vi "Phasor Compute 1-Exp Gate Array v2.vi"(8 "Error In":errorcluster, 9 "Gates Definitions":T3={"First Gate: t1"=0.0, "Gate Width: W"=0.0, "Gate Step: d"=0.0, "# Gates: G"=0.0, "Use Gate Center"=FALSE, "Frames/Image: F"=50, "Gates/Frame: L"=0, "Bits/Frame: q"=0, "Multiplicity: p"=0, "Gate Type"=enum."Square", "Gate Edge s"=4.0, "Gate Top Slope"=4.0, "Reversed Sawtooth?"=FALSE, "Computation"=FALSE, "User-defined Gate"={"X Array"=[], "Y Array"=[]}, "Tolerance"=50.0, "Integration"=enum."Item 0", "# Steps"=50.0, "Type of User-defined Function"=enum."Gate"}, 11 "Decay Definition":T1={"offset: t0"=0.0, "period: T"=0.0, "lifetime: tau"=0.0, "Incident Signal: I"=0.5, "Normalized Decays"=FALSE, "IRF Model"=enum."Dirac", "IRF Parameter 1"=0.0, "Poisson Signal"=FALSE}) -> (0 "Error Out":errorcluster, 1 "Gate Image Array":ext[](array[numeric]), 3 "t Array":ext[](array[numeric]), 4 "Small Gate Values?":bool, 6 "CPU (s)":dbl)   [LabVIEW 2021, in "Phasor.lvlib"]
uses:
  Phasor.lvlib
  Phasor Gate Definitions.ctl
  Phasor Gate Type.ctl
  Graphs/XY Graph/XY Plot Data.ctl
  Phasor Decay Definiton.ctl
  Phasor IRF Model.ctl
  Phasor Photon-Counting Saturation Parameters.ctl
  Arrays/Linear Ramp End Options.ctl
  Phasor Gate & Decay Parameters.ctl
  c327f329-df48-4cbd-af17-0505137efb44.vi
  19793270-9f6f-421c-b0b4-4a6df58db2d8.vi
  bce56a49-f57b-428e-8cfb-829b6e224b2d.vi
  9dc9122e-8396-4e29-9b52-206296392f6e.vi
  09e65239-3f09-4922-a97b-00e12ebb298a.vi
  a4873a35-ead0-464d-8454-7d3b7b3dc21e.vi
  430a8be0-ec63-490d-ae91-6adec514d333.vi
  bfad809a-910b-4a1f-913e-0342548baa46.vi
  822bd012-03ef-446a-9035-c62730970759.vi
  9329e439-e603-4ca8-9979-680bb8b82628.vi
  12aa5bdc-9085-4c22-9899-1a2d30a0f259.vi
  2b2e435f-01ea-4379-bbb3-bd43ea243b44.vi
  e19b1486-ca4b-43fe-9b82-4ecd58cc5538.vi
  9dc9122e-8396-4e29-9b52-206296392f6e.vi/8a80743f-1319-44c8-96b0-3ef8fc688731.vi
  9dc9122e-8396-4e29-9b52-206296392f6e.vi/931f4f8f-d8c6-4056-833f-5c8fe97b24b9.vi
  09e65239-3f09-4922-a97b-00e12ebb298a.vi/8a80743f-1319-44c8-96b0-3ef8fc688731.vi
  09e65239-3f09-4922-a97b-00e12ebb298a.vi/931f4f8f-d8c6-4056-833f-5c8fe97b24b9.vi
  430a8be0-ec63-490d-ae91-6adec514d333.vi/8a80743f-1319-44c8-96b0-3ef8fc688731.vi
  430a8be0-ec63-490d-ae91-6adec514d333.vi/931f4f8f-d8c6-4056-833f-5c8fe97b24b9.vi
  9329e439-e603-4ca8-9979-680bb8b82628.vi/8a80743f-1319-44c8-96b0-3ef8fc688731.vi
  9329e439-e603-4ca8-9979-680bb8b82628.vi/931f4f8f-d8c6-4056-833f-5c8fe97b24b9.vi
  2b2e435f-01ea-4379-bbb3-bd43ea243b44.vi/8a80743f-1319-44c8-96b0-3ef8fc688731.vi
  2b2e435f-01ea-4379-bbb3-bd43ea243b44.vi/931f4f8f-d8c6-4056-833f-5c8fe97b24b9.vi
  Phasor Abort Parallel Computation.vi
  Arrays/Arrays.lvlib
  Graphs/XY Graph/XY Graph Add-Ons.lvlib
  Time/Time.lvlib
panel:
  out "XY Graph":cluster{ext[], ext[]}[](graph)
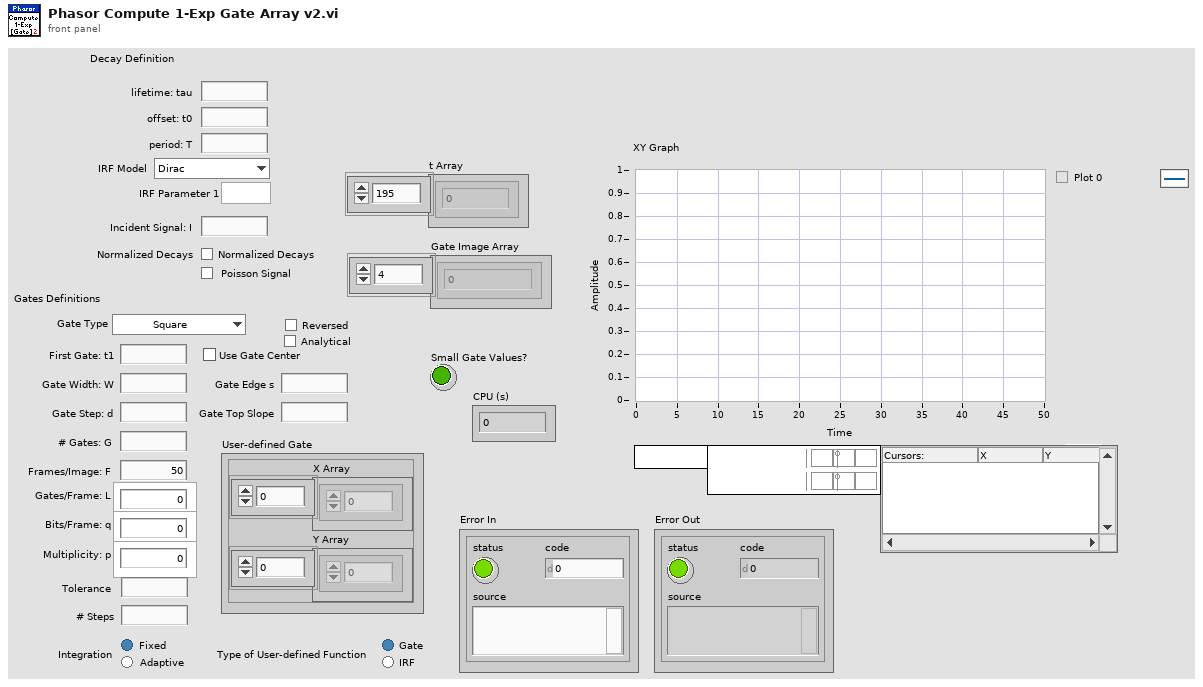
[diagram p1: front panel]
types:
  T1 = typedef "Phasor.lvlib/Phasor Decay Definiton.ctl" = cluster{"offset: t0":ext, "period: T":ext, "lifetime: tau":ext, "Incident Signal: I":ext, "Normalized Decays":bool, "IRF Model":T2, "IRF Parameter 1":ext, "Poisson Signal":bool}
  T2 = typedef "Phasor.lvlib/Phasor IRF Model.ctl" = enum16{"Dirac", "Exponential"}
  T3 = typedef "Phasor.lvlib/Phasor Gate Definitions.ctl" = cluster{"First Gate: t1":ext, "Gate Width: W":ext, "Gate Step: d":ext, "# Gates: G":ext, "Use Gate Center":bool, "Frames/Image: F":i32, "Gates/Frame: L":i32, "Bits/Frame: q":i32, "Multiplicity: p":i32, "Gate Type":T4, "Gate Edge s":ext, "Gate Top Slope":ext, "Reversed Sawtooth?":bool, "Computation":bool, "User-defined Gate":T5, "Tolerance":ext, "Integration":enum32{"Item 0", "Item 1"}, "# Steps":ext, "Type of User-defined Function":enum32{"Gate", "IRF"}}
  T4 = typedef "Phasor.lvlib/Phasor Gate Type.ctl" = enum16{"Square", "Finite Edge Square", "Finite Edge, Tilted Top Square", "Triangle", "Sawtooth", "User-defined"}
  T5 = typedef "XY Graph Add-Ons.lvlib/XY Plot Data.ctl" = cluster{"X Array":dbl[], "Y Array":dbl[]}
  T6 = typedef "Phasor.lvlib/Phasor Photon-Counting Saturation Parameters.ctl" = cluster{"Frames/Image: F":i32, "Gates/Frame: L":i32, "Multiplicity: p":i32, "Bits/Frame: q":i32}
  T7 = typedef "Phasor.lvlib/Phasor Gate & Decay Parameters.ctl" = cluster{"W":dbl, "T":dbl, "tau":dbl, "t_0":dbl, "Gate Type":T4, "t_i":dbl, "sR":dbl, "sF":dbl, "s":dbl, "Reversed Sawtooth":bool, "IRF Model":T2, "IRF Parameter 1":dbl, "User-defined Gate":T5, "Type of User-defined Function":enum32{"Gate", "IRF"}, "A":dbl}
  T8 = typedef "Arrays.lvlib/Linear Ramp End Options.ctl" = enum16{"Include Min/Exclude Max", "Exclude Min/Include Max", "Include Both Ends", "Exclude Both Ends"}
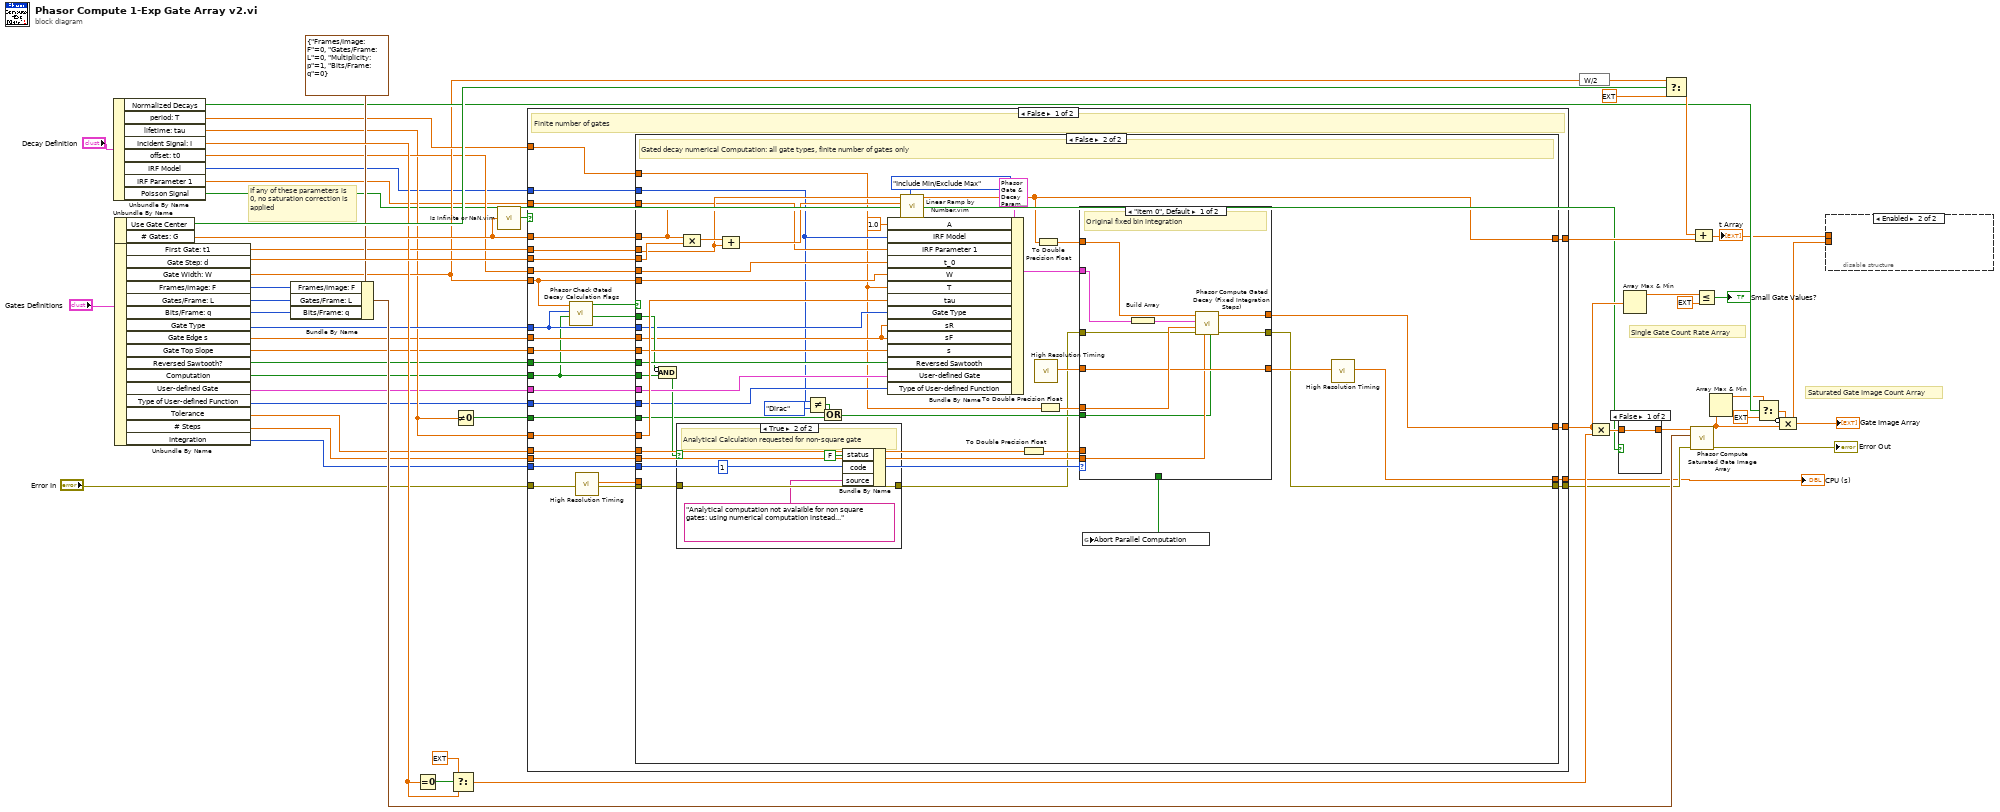
[diagram p0: block diagram]
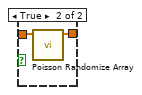
[diagram p2: hidden frame]
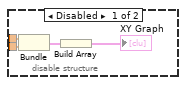
[diagram p3: hidden frame]
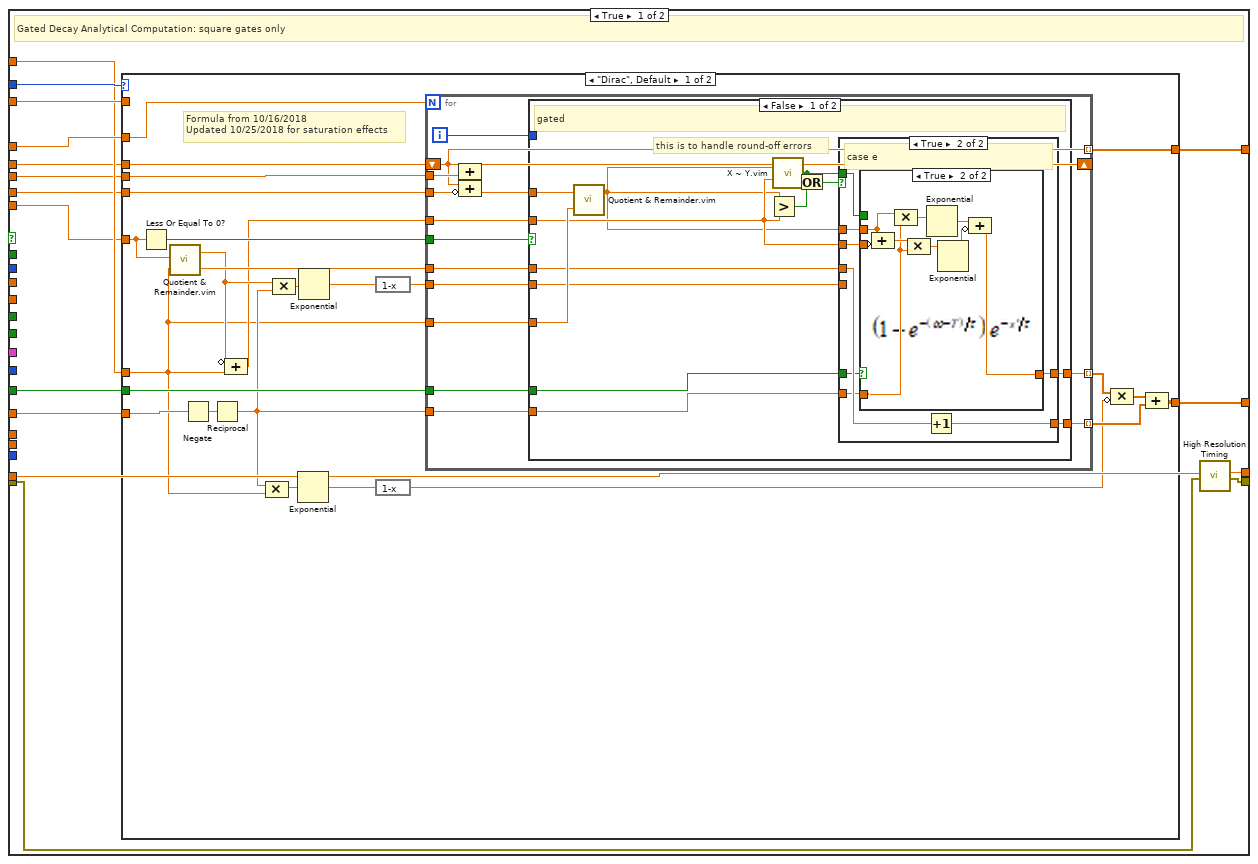
[diagram p4: hidden frame]
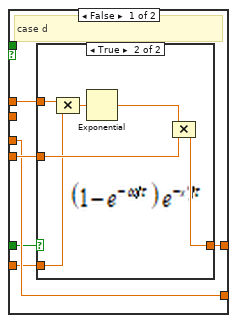
[diagram p5: hidden frame]
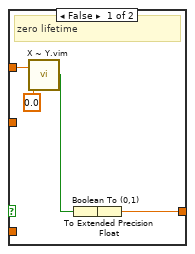
[diagram p6: hidden frame]
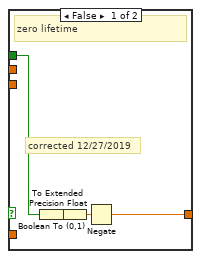
[diagram p7: hidden frame]
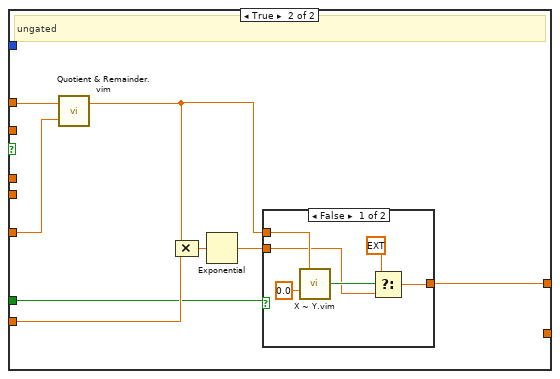
[diagram p8: hidden frame]
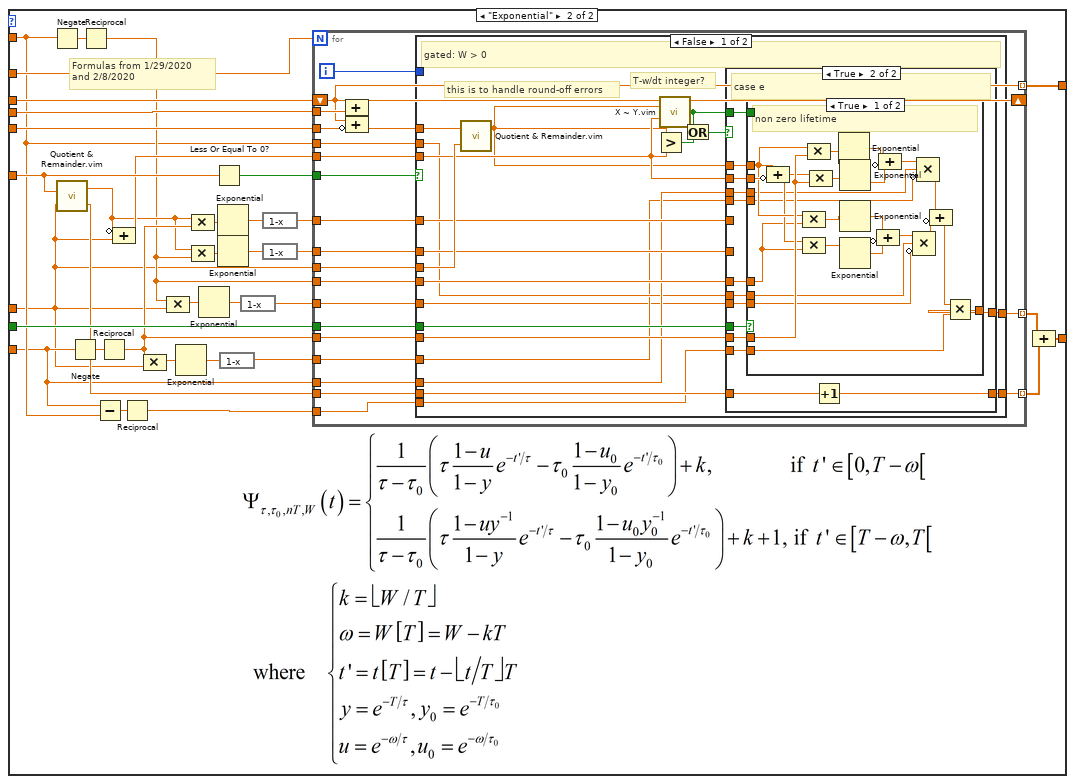
[diagram p10: hidden frame]
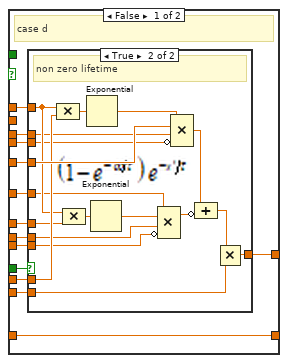
[diagram p11: hidden frame]
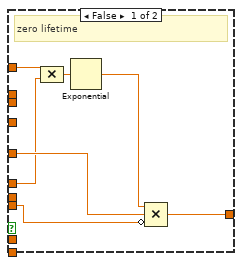
[diagram p12: hidden frame]
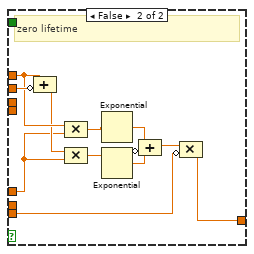
[diagram p13: hidden frame]
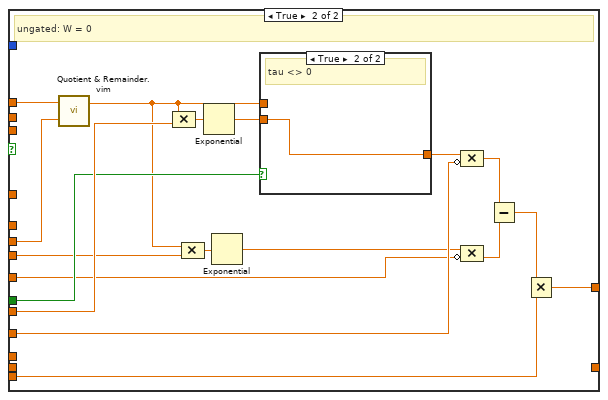
[diagram p14: hidden frame]
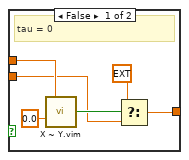
[diagram p15: hidden frame]
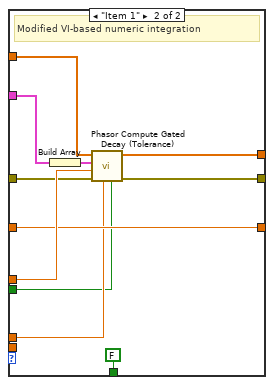
[diagram p16: hidden frame]
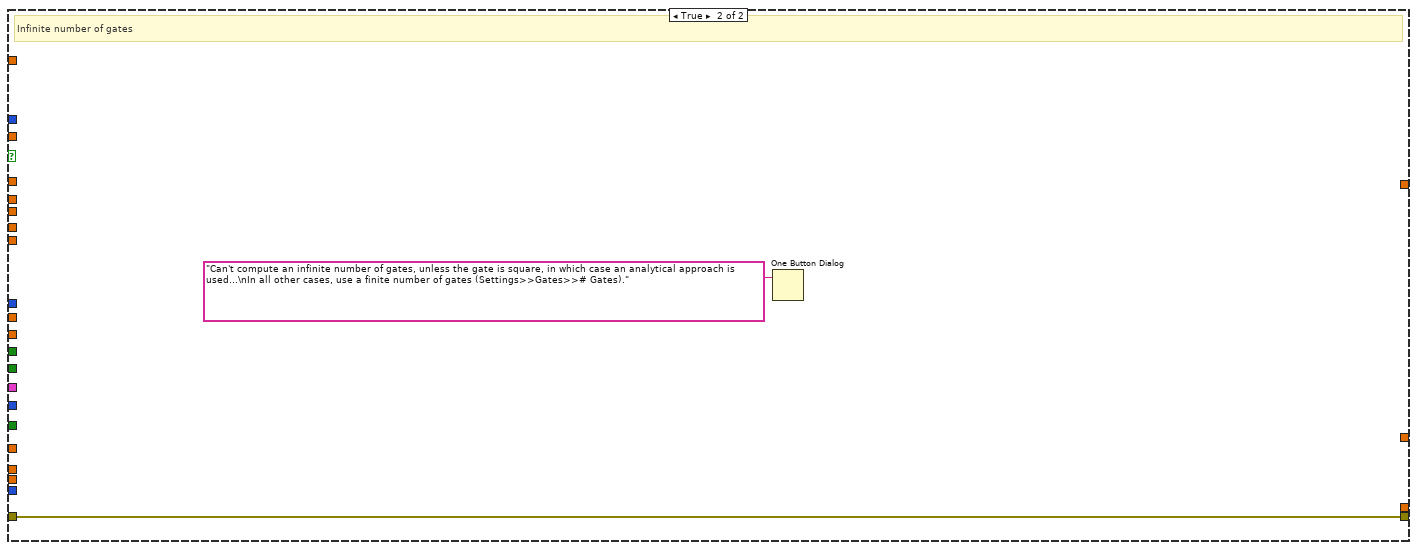
[diagram p18: hidden frame]
diagram:
  # "If any of these parameters is 0, no saturation correction is applied"
  # "Saturated Gate Image Count Array"
  # "Single Gate Count Rate Array"
  n1 = Unbundle By Name("Decay Definition") -> ("Normalized Decays"=w36:bool, "period: T"=w32:ext, "lifetime: tau"=w23:ext, "Incident Signal: I"=w44:ext, "offset: t0"=w27:ext, "IRF Model"=w11:T2, "IRF Parameter 1"=w10:ext, "Poisson Signal"=w1:bool)
  n2 = Unbundle By Name("Gates Definitions") -> ("Use Gate Center"=w48:bool, "# Gates: G"=w49:ext)
  n3 = Unbundle By Name("Gates Definitions") -> ("First Gate: t1"=w33:ext, "Gate Step: d"=w55:ext, "Gate Width: W"=w28:ext, "Frames/Image: F"=w43:i32, "Gates/Frame: L"=w42:i32, "Bits/Frame: q"=w41:i32, "Gate Type"=w26:T4, "Gate Edge s"=w21:ext, "Gate Top Slope"=w20:ext, "Reversed Sawtooth?"=w16:bool, "Computation"=w12:bool, "User-defined Gate"=w9:T5, "Type of User-defined Function"=w4:enum32{"Gate", "IRF"}, "Tolerance"=w8:ext, "# Steps"=w5:ext, "Integration"=w6:enum32{"Item 0", "Item 1"})
  n4 = Bundle By Name(cluster=T6 {"Frames/Image: F"=0, "Gates/Frame: L"=0, "Multiplicity: p"=1, "Bits/Frame: q"=0} ("Saturation Parameters"), "Frames/Image: F"=w43, "Gates/Frame: L"=w42, "Bits/Frame: q"=w41) -> (w40:T6)
  n5 = Equal To 0?(x=w44) -> (x = 0?=w45:bool)
  n6 = Select(t=ext 1.0, s=w45, f=w44) -> (s? t:f=w46:ext)
  n7 = Not Equal To 0?(x=w23) -> (x != 0?=w22:bool)
  n8 = call "Is Infinite or NaN.vim"("Number"=w49) -> ("Is NaN or Inf?"=w13:bool)  [unwired: 8 in]
  n9 = case shown="False" w13 {
    tunnel: w26 -> [w70 _]
    tunnel: w33 -> [w84 _]
    tunnel: w55 -> [w83 _]
    tunnel: w27 -> [w82 _]
    tunnel: w32 -> [w81 _]
    tunnel: w23 -> [w80 _]
    tunnel: [w79 _] -> w25
    tunnel: [w78 _] -> w24
    tunnel: w22 -> [w77 _]
    tunnel: w21 -> [w76 _]
    tunnel: w20 -> [w75 _]
    tunnel: w16 -> [w74 _]
    tunnel: w49 -> [w73 _]
    tunnel: w28 -> [w63 _]
    tunnel: "Error In" -> [w71 w467]
    tunnel: [w72 w467] -> w14
    tunnel: w12 -> [w65 _]
    tunnel: w11 -> [w69 _]
    tunnel: w10 -> [w68 _]
    tunnel: w9 -> [w67 _]
    tunnel: w8 -> [w66 _]
    tunnel: [w62 _] -> w7
    tunnel: w6 -> [w59 _]
    tunnel: w5 -> [w58 _]
    tunnel: w4 -> [w57 _]
    frame False {
      # "Finite number of gates"
      n10 = call "Phasor Check Gated Decay Calculation Flags.vi"("Analytical Computation?"=w65, "Gate/IRF Type"=w70, "Gate Width: W"=w63) -> ("Square Gate?"=w56:bool, "Analytical?"=w64:bool)  [unwired: 7 in]
      n11 = call "High Resolution Timing.vi"("Error In"=w71) -> ("elapsed (relative) seconds"=w60:dbl, "Error Out"=w61:errorcluster)  [unwired: 16 in, 1 out]
      n12 = case shown="False" w64 {
        tunnel: w73 -> [w94 w435]
        tunnel: w84 -> [w88 w432]
        tunnel: w83 -> [w89 w433]
        tunnel: w82 -> [w90 w415]
        tunnel: w63 -> [w91 w411]
        tunnel: w81 -> [w92 w402]
        tunnel: w80 -> [w93 w434]
        tunnel: [w100 w430] -> w78
        tunnel: [w99 w431] -> w79
        tunnel: w77 -> [w98 w416]
        tunnel: w76 -> [_ w413]
        tunnel: w75 -> [_ w429]
        tunnel: w74 -> [_ w428]
        tunnel: [w87 w397] -> w72
        tunnel: w61 -> [w97 w424]
        tunnel: w70 -> [_ w412]
        tunnel: w69 -> [w96 w404]
        tunnel: w68 -> [w95 w427]
        tunnel: w67 -> [_ w426]
        tunnel: w66 -> [_ w425]
        tunnel: w65 -> [_ w423]
        tunnel: w56 -> [_ w422]
        tunnel: [w85 w406] -> w62
        tunnel: w60 -> [w86 _]
        tunnel: w59 -> [_ w417]
        tunnel: w58 -> [_ w414]
        tunnel: w57 -> [_ w410]
        frame True {
          # "Gated Decay Analytical Computation: square gates only"
          n13 = case shown="\"Dirac\", Default" w96 {
            tunnel: w94 -> [w125 w241]
            tunnel: w88 -> [w124 w240]
            tunnel: w89 -> [w123 w239]
            tunnel: w90 -> [w122 w238]
            tunnel: w91 -> [w121 w237]
            tunnel: w92 -> [w101 w207]
            tunnel: w93 -> [w120 w208]
            tunnel: [w119 w236] -> w100
            tunnel: [w118 w235] -> w99
            tunnel: w98 -> [w117 w234]
            tunnel: w95 -> [_ w209]
            frame "Dirac", Default {
              # "Formula from 10/16/2018\nUpdated 10/25/2018 for saturation effects"
              n14 = Less Or Equal To 0?(x=w121) -> (x <= 0?=w106:bool)
              n15 = call "Quotient & Remainder.vim"("y"=w101, "x"=w121) -> ("E(x/y)"=w109:ext, "x - E(x/y)y"=w105:ext)
              n16 = Negate(x=w120) -> (-x=w114:ext)
              n17 = Reciprocal(x=w114) -> (1/x=w104:ext)
              n18 = Compound Arithmetic op=ADD(invert w105, w101) -> (w102:ext)
              n19 = Compound Arithmetic op=MULTIPLY(w104, w101) -> (w113:ext)
              n20 = Compound Arithmetic op=MULTIPLY(w105, w104) -> (w112:ext)
              n21 = Exponential(1:w113) -> (0:w108:ext)
              n22 = Exponential(1:w112) -> (0:w111:ext)
              n23 = expression code="1-x"(w111) -> (w110:ext)
              n24 = expression code="1-x"(w108) -> (w107:ext)
              n25 = for {
                N: w125 -> [_]
                tunnel: w123 -> [w140]
                tunnel: w122 -> [w138]
                tunnel: w101 -> [w136]
                tunnel: w104 -> [w135]
                shift-right: [w139] -> _
                shift-left: w124 -> [w131]
                tunnel: [w131] -> w119 mode=indexing
                tunnel: w110 -> [w134]
                tunnel: w109 -> [w133]
                tunnel: [w127] -> w103 mode=indexing
                tunnel: [w132] -> w116 mode=indexing
                tunnel: w106 -> [w130]
                tunnel: w102 -> [w129]
                tunnel: w117 -> [w128]
                i -> [w126]
                n26 = Compound Arithmetic op=ADD(w131, w140) -> (w139:ext)
                n27 = Compound Arithmetic op=ADD(w131, invert w138) -> (w137:ext)
                n28 = case shown="False" w130 {
                  tunnel: w137 -> [w153 w192]
                  tunnel: w136 -> [w152 w199]
                  tunnel: w135 -> [w146 w198]
                  tunnel: w134 -> [w151 _]
                  tunnel: [w150 w196] -> w127
                  tunnel: w133 -> [w149 _]
                  tunnel: [w148 _] -> w132
                  tunnel: w129 -> [w144 _]
                  tunnel: w128 -> [w145 w193]
                  tunnel: w126 -> [_ _]
                  frame False {
                    # "this is to handle round-off errors"
                    # "gated"
                    n29 = call "Quotient & Remainder.vim"("y"=w152, "x"=w153) -> ("x - E(x/y)y"=w141:ext)  [unwired: 1 out]
                    n30 = Greater?(x=w141, y=w144) -> (0:w147:bool)
                    n31 = call "X ~ Y.vim"("X"=w141, "Y"=w144) -> ("X ~= Y?"=w143:bool)  [unwired: 13 in]
                    n32 = Or(x=w143, y=w147) -> (x .or. y?=w142:bool)
                    n33 = case shown="True" w142 {
                      tunnel: w151 -> [w159 _]
                      tunnel: [w158 w174] -> w150
                      tunnel: w149 -> [w157 w178]
                      tunnel: [w157 w177] -> w148
                      tunnel: w141 -> [w156 w176]
                      tunnel: w146 -> [w155 w175]
                      tunnel: w144 -> [_ w173]
                      tunnel: w145 -> [w154 w172]
                      tunnel: w143 -> [_ w171]
                      frame False {
                        # "case d"
                        n34 = case shown="True" w154 {
                          tunnel: w159 -> [_ w170]
                          tunnel: [w163 w169] -> w158
                          tunnel: w156 -> [w162 w167]
                          tunnel: w155 -> [_ w166]
                          frame False {
                            # "zero lifetime"
                            n35 = call "X ~ Y.vim"("X"=w162, "Y"=0.0) -> ("X ~= Y?"=w160:bool)  [unwired: 13 in]
                            n36 = Boolean To (0,1)(Boolean=w160) -> (0, 1=w164:i16)
                            n37 = To Extended Precision Float(1:w164) -> (0:w163:ext)
                          }
                          frame True {
                            n38 = Compound Arithmetic op=MULTIPLY(w167, w166) -> (w168:ext)
                            n39 = Exponential(1:w168) -> (0:w165:ext)
                            n40 = Compound Arithmetic op=MULTIPLY(w165, w170) -> (w169:ext)
                          }
                        }
                      }
                      frame True {
                        # "case e"
                        n41 = case shown="True" w172 {
                          tunnel: w176 -> [_ w189]
                          tunnel: w175 -> [_ w188]
                          tunnel: [w180 w184] -> w174
                          tunnel: w173 -> [_ w183]
                          tunnel: w171 -> [w179 _]
                          frame False {
                            # "corrected 12/27/2019"
                            # "zero lifetime"
                            n42 = Boolean To (0,1)(Boolean=w179) -> (0, 1=w182:i16)
                            n43 = To Extended Precision Float(1:w182) -> (0:w181:ext)
                            n44 = Negate(x=w181) -> (-x=w180:ext)
                          }
                          frame True {
                            n45 = Compound Arithmetic op=ADD(w189, invert w183) -> (w191:ext)
                            n46 = Compound Arithmetic op=MULTIPLY(w189, w188) -> (w187:ext)
                            n47 = Compound Arithmetic op=MULTIPLY(w191, w188) -> (w190:ext)
                            n48 = Exponential(1:w187) -> (0:w186:ext)
                            n49 = Exponential(1:w190) -> (0:w185:ext)
                            n50 = Compound Arithmetic op=ADD(w186, invert w185) -> (w184:ext)
                          }
                        }
                        n51 = Increment(x=w178) -> (x+1=w177:ext)
                      }
                    }
                  }
                  frame True {
                    # "ungated"
                    n52 = call "Quotient & Remainder.vim"("y"=w199, "x"=w192) -> ("x - E(x/y)y"=w195:ext)  [unwired: 1 out]
                    n53 = Compound Arithmetic op=MULTIPLY(w195, w198) -> (w197:ext)
                    n54 = Exponential(1:w197) -> (0:w194:ext)
                    n55 = case shown="False" w193 {
                      tunnel: [w205 w206] -> w196
                      tunnel: w195 -> [w204 _]
                      tunnel: w194 -> [w200 w206]
                      frame False {
                        n56 = call "X ~ Y.vim"("X"=w204, "Y"=0.0) -> ("X ~= Y?"=w202:bool)  [unwired: 13 in]
                        n57 = Select(t=ext 1.0 ("f"), s=w202, f=w200) -> (s? t:f=w205:ext)
                      }
                      frame True {
                      }
                    }
                  }
                }
              }
              n58 = Compound Arithmetic op=MULTIPLY(w103, invert w107) -> (w115:ext[])
              n59 = Compound Arithmetic op=ADD(w115, w116) -> (w118:ext[])
            }
            frame "Exponential" {
              # "Formulas from 1/29/2020\nand 2/8/2020"
              n60 = Negate(x=w209) -> (-x=w222:ext)
              n61 = call "Quotient & Remainder.vim"("y"=w207, "x"=w237) -> ("E(x/y)"=w227:ext, "x - E(x/y)y"=w214:ext)
              n62 = Negate(x=w208) -> (-x=w232:ext)
              n63 = Reciprocal(x=w222) -> (1/x=w213:ext)
              n64 = Subtract(x=w208, y=w209) -> (x-y=w211:ext)
              n65 = Reciprocal(x=w232) -> (1/x=w224:ext)
              n66 = Compound Arithmetic op=ADD(invert w214, w207) -> (w223:ext)
              n67 = Reciprocal(x=w211) -> (1/x=w210:ext)
              n68 = Compound Arithmetic op=MULTIPLY(w224, w207) -> (w231:ext)
              n69 = Compound Arithmetic op=MULTIPLY(w213, w207) -> (w218:ext)
              n70 = Exponential(1:w231) -> (0:w226:ext)
              n71 = Compound Arithmetic op=MULTIPLY(w214, w224) -> (w230:ext)
              n72 = Compound Arithmetic op=MULTIPLY(w214, w213) -> (w215:ext)
              n73 = Exponential(1:w218) -> (0:w219:ext)
              n74 = Less Or Equal To 0?(x=w237) -> (x <= 0?=w225:bool)
              n75 = Exponential(1:w230) -> (0:w229:ext)
              n76 = Exponential(1:w215) -> (0:w216:ext)
              n77 = expression code="1-x"(w226) -> (w221:ext)
              n78 = expression code="1-x"(w219) -> (w217:ext)
              n79 = expression code="1-x"(w229) -> (w228:ext)
              n80 = expression code="1-x"(w216) -> (w212:ext)
              n81 = for {
                N: w241 -> [_]
                tunnel: w239 -> [w263]
                tunnel: w238 -> [w261]
                tunnel: w207 -> [w259]
                tunnel: w224 -> [w258]
                shift-right: [w262] -> _
                shift-left: w240 -> [w255]
                tunnel: [w255] -> w236 mode=indexing
                tunnel: w228 -> [w257]
                tunnel: w227 -> [w242]
                tunnel: [w244] -> w220 mode=indexing
                tunnel: [w256] -> w233 mode=indexing
                tunnel: w225 -> [w254]
                tunnel: w223 -> [w253]
                tunnel: w234 -> [w252]
                tunnel: w213 -> [w250]
                tunnel: w221 -> [w245]
                tunnel: w217 -> [w249]
                tunnel: w212 -> [w248]
                tunnel: w210 -> [w243]
                tunnel: w209 -> [w247]
                tunnel: w208 -> [w246]
                i -> [w251]
                n82 = Compound Arithmetic op=ADD(w255, w263) -> (w262:ext)
                n83 = Compound Arithmetic op=ADD(w255, invert w261) -> (w260:ext)
                n84 = case shown="False" w254 {
                  tunnel: w260 -> [w283 w388]
                  tunnel: w259 -> [w282 w387]
                  tunnel: w258 -> [w277 w386]
                  tunnel: w257 -> [w281 _]
                  tunnel: w242 -> [w280 _]
                  tunnel: [w279 _] -> w256
                  tunnel: w253 -> [w275 _]
                  tunnel: w252 -> [w276 w383]
                  tunnel: w251 -> [_ _]
                  tunnel: w250 -> [w271 w379]
                  tunnel: w249 -> [w265 w376]
                  tunnel: w248 -> [w270 _]
                  tunnel: w247 -> [w268 _]
                  tunnel: w246 -> [w269 _]
                  tunnel: w245 -> [w267 w381]
                  tunnel: [w266 w371] -> w244
                  tunnel: w243 -> [w264 w372]
                  frame False {
                    # "T-w/dt integer?"
                    # "this is to handle round-off errors"
                    # "gated: W > 0"
                    n85 = call "Quotient & Remainder.vim"("y"=w282, "x"=w283) -> ("x - E(x/y)y"=w272:ext)  [unwired: 1 out]
                    n86 = Greater?(x=w272, y=w275) -> (0:w278:bool)
                    n87 = call "X ~ Y.vim"("X"=w272, "Y"=w275) -> ("X ~= Y?"=w274:bool)  [unwired: 13 in]
                    n88 = Or(x=w274, y=w278) -> (x .or. y?=w273:bool)
                    n89 = case shown="True" w273 {
                      tunnel: w281 -> [w296 _]
                      tunnel: [w295 w331] -> w266
                      tunnel: w280 -> [w294 w335]
                      tunnel: [w294 w334] -> w279
                      tunnel: w272 -> [w293 w333]
                      tunnel: w277 -> [w292 w332]
                      tunnel: w275 -> [_ w330]
                      tunnel: w276 -> [w291 w329]
                      tunnel: w274 -> [_ w328]
                      tunnel: w271 -> [w290 w327]
                      tunnel: w270 -> [w289 _]
                      tunnel: w269 -> [w288 w326]
                      tunnel: w268 -> [w287 w325]
                      tunnel: w267 -> [w286 w324]
                      tunnel: w265 -> [w285 w323]
                      tunnel: w264 -> [w284 w322]
                      frame False {
                        # "case d"
                        n90 = case shown="True" w291 {
                          tunnel: w296 -> [_ w321]
                          tunnel: [w301 w305] -> w295
                          tunnel: w293 -> [w299 w316]
                          tunnel: w292 -> [_ w318]
                          tunnel: w290 -> [w298 w315]
                          tunnel: w289 -> [w303 w313]
                          tunnel: w288 -> [_ w311]
                          tunnel: w287 -> [_ w310]
                          tunnel: w286 -> [_ w309]
                          tunnel: w285 -> [w302 w308]
                          tunnel: w284 -> [_ w304]
                          frame False {
                            # "zero lifetime"
                            n91 = Compound Arithmetic op=MULTIPLY(w299, w298) -> (w300:ext)
                            n92 = Exponential(1:w300) -> (0:w297:ext)
                            n93 = Compound Arithmetic op=MULTIPLY(w297, w303, invert w302) -> (w301:ext)
                          }
                          frame True {
                            # "non zero lifetime"
                            n94 = Compound Arithmetic op=MULTIPLY(w316, w318) -> (w319:ext)
                            n95 = Compound Arithmetic op=MULTIPLY(w316, w315) -> (w314:ext)
                            n96 = Exponential(1:w319) -> (0:w317:ext)
                            n97 = Exponential(1:w314) -> (0:w312:ext)
                            n98 = Compound Arithmetic op=MULTIPLY(w313, w312, w310, invert w308) -> (w306:ext)
                            n99 = Compound Arithmetic op=MULTIPLY(w317, w321, w311, invert w309) -> (w320:ext)
                            n100 = Compound Arithmetic op=ADD(w320, invert w306) -> (w307:ext)
                            n101 = Multiply(x=w307, y=w304) -> (x*y=w305:ext)
                          }
                        }
                      }
                      frame True {
                        # "case e"
                        n102 = case shown="True" w329 {
                          tunnel: w333 -> [w352 w369]
                          tunnel: w332 -> [w358 _]
                          tunnel: [w337 w360] -> w331
                          tunnel: w330 -> [w353 w370]
                          tunnel: w328 -> [_ _]
                          tunnel: w327 -> [w350 w367]
                          tunnel: w326 -> [w344 _]
                          tunnel: w325 -> [w342 _]
                          tunnel: w324 -> [w341 _]
                          tunnel: w323 -> [w340 w361]
                          tunnel: w322 -> [w336 _]
                          frame True {
                            # "non zero lifetime"
                            n103 = Compound Arithmetic op=ADD(w352, invert w353) -> (w351:ext)
                            n104 = Compound Arithmetic op=MULTIPLY(w352, w350) -> (w349:ext)
                            n105 = Compound Arithmetic op=MULTIPLY(w351, w350) -> (w348:ext)
                            n106 = Compound Arithmetic op=MULTIPLY(w352, w358) -> (w357:ext)
                            n107 = Compound Arithmetic op=MULTIPLY(w351, w358) -> (w359:ext)
                            n108 = Exponential(1:w357) -> (0:w356:ext)
                            n109 = Exponential(1:w359) -> (0:w355:ext)
                            n110 = Exponential(1:w349) -> (0:w347:ext)
                            n111 = Exponential(1:w348) -> (0:w346:ext)
                            n112 = Compound Arithmetic op=ADD(w347, invert w346) -> (w343:ext)
                            n113 = Compound Arithmetic op=ADD(w356, invert w355) -> (w354:ext)
                            n114 = Compound Arithmetic op=MULTIPLY(w343, w342, invert w340) -> (w338:ext)
                            n115 = Compound Arithmetic op=MULTIPLY(w354, w344, invert w341) -> (w345:ext)
                            n116 = Compound Arithmetic op=ADD(w345, invert w338) -> (w339:ext)
                            n117 = Multiply(x=w339, y=w336) -> (x*y=w337:ext)
                          }
                          frame False {
                            # "zero lifetime"
                            n118 = Compound Arithmetic op=ADD(w369, invert w370) -> (w368:ext)
                            n119 = Compound Arithmetic op=MULTIPLY(w369, w367) -> (w366:ext)
                            n120 = Compound Arithmetic op=MULTIPLY(w368, w367) -> (w365:ext)
                            n121 = Exponential(1:w366) -> (0:w364:ext)
                            n122 = Exponential(1:w365) -> (0:w363:ext)
                            n123 = Compound Arithmetic op=ADD(w364, invert w363) -> (w362:ext)
                            n124 = Compound Arithmetic op=MULTIPLY(w362, invert w361) -> (w360:ext)
                          }
                        }
                        n125 = Increment(x=w335) -> (x+1=w334:ext)
                      }
                    }
                  }
                  frame True {
                    # "ungated: W = 0"
                    n126 = call "Quotient & Remainder.vim"("y"=w387, "x"=w388) -> ("x - E(x/y)y"=w380:ext)  [unwired: 1 out]
                    n127 = Compound Arithmetic op=MULTIPLY(w380, w386) -> (w385:ext)
                    n128 = Compound Arithmetic op=MULTIPLY(w380, w379) -> (w378:ext)
                    n129 = Exponential(1:w385) -> (0:w384:ext)
                    n130 = Exponential(1:w378) -> (0:w377:ext)
                    n131 = case shown="True" w383 {
                      tunnel: [w394 w395] -> w382
                      tunnel: w380 -> [w393 _]
                      tunnel: w384 -> [w389 w395]
                      frame False {
                        # "tau = 0"
                        n132 = call "X ~ Y.vim"("X"=w393, "Y"=0.0) -> ("X ~= Y?"=w391:bool)  [unwired: 13 in]
                        n133 = Select(t=ext 1.0 ("f"), s=w391, f=w389) -> (s? t:f=w394:ext)
                      }
                      frame True {
                        # "tau <> 0"
                      }
                    }
                    n134 = Compound Arithmetic op=MULTIPLY(w382, invert w381) -> (w375:ext)
                    n135 = Compound Arithmetic op=MULTIPLY(w377, invert w376) -> (w374:ext)
                    n136 = Subtract(x=w375, y=w374) -> (x-y=w373:ext)
                    n137 = Multiply(x=w373, y=w372) -> (x*y=w371:ext)
                  }
                }
              }
              n138 = Compound Arithmetic op=ADD(w220, w233) -> (w235:ext[])
            }
          }
          n139 = call "High Resolution Timing.vi"("relative seconds (NaN)"=w86, "Error In"=w97) -> ("elapsed (relative) seconds"=w85:dbl, "Error Out"=w87:errorcluster)  [unwired: 15 in, 1 out]
        }
        frame False {
          # "Gated decay numerical Computation: all gate types, finite number of gates only"
          n140 = Compound Arithmetic op=AND(invert w422, w423) -> (w421:bool)
          n141 = case shown="True" w421 {
            tunnel: w424 -> [w460 w465]
            tunnel: [w460 w464] -> w398
            frame False {
            }
            frame True {
              # "Analytical Calculation requested for non-square gate"
              n142 = Bundle By Name(cluster=w465, "status"=FALSE, "code"=1 ("error code (0)"), "source"="Analytical computation not avalaible for non square gates: using numerical computation instead..." ("message")) -> (w464:errorcluster)
            }
          }
          n143 = Compound Arithmetic op=MULTIPLY(w435, w433) -> (w438:ext)
          n144 = Compound Arithmetic op=ADD(w438, w432) -> (w437:ext)
          n145 = Not Equal?(x=w404, y=Phasor_IRF_Model."Dirac" ("IRF Model")) -> (x != y?=w401:bool)
          n146 = Compound Arithmetic op=OR(w401, w416) -> (w400:bool)
          n147 = Bundle By Name(cluster=T7 {"W"=0.0, "T"=0.0, "tau"=0.0, "t_0"=0.0, "Gate Type"=enum."Square", "t_i"=0.0, "sR"=0.0, "sF"=0.0, "s"=0.0, "Reversed Sawtooth"=FALSE, "IRF Model"=enum."Dirac", "IRF Parameter 1"=0.0, "User-defined Gate"={"X Array"=[], "Y Array"=[]}, "Type of User-defined Function"=enum."Gate", "A"=0.0} ("Gate & Decay Parameters"), "A"=1.0, "IRF Model"=w404, "IRF Parameter 1"=w427, "t_0"=w415, "W"=w411, "T"=w402, "tau"=w434, "Gate Type"=w412, "sR"=w413, "sF"=w413, "s"=w429, "Reversed Sawtooth"=w428, "User-defined Gate"=w426, "Type of User-defined Function"=w410) -> (w419:T7)
          n148 = call "Linear Ramp by Number.vim"("Options"=Linear_Ramp_End_Options."Include Min/Exclude Max", "# Steps (1)"=w435, "End (1)"=w437, "Start (0)"=w432) -> ("Ramp"=w430:ext[])  [unwired: 5 in, 2 out]
          n149 = To Double Precision Float(number=w425) -> (double precision float=w408:dbl)
          n150 = call "High Resolution Timing.vi"() -> ("elapsed (relative) seconds"=w407:dbl)  [unwired: 17 in, 2 out]
          n151 = To Double Precision Float(number=w430) -> (double precision float=w418:dbl[])
          n152 = To Double Precision Float(number=w402) -> (double precision float=w409:dbl)
          n153 = case shown="\"Item 0\", Default" w417 {
            tunnel: [w448 w457] -> w431
            tunnel: w408 -> [_ w453]
            tunnel: w419 -> [w447 w458]
            tunnel: [w443 w451] -> w397
            tunnel: w418 -> [w446 w459]
            tunnel: w409 -> [w445 w456]
            tunnel: w414 -> [w442 _]
            tunnel: w407 -> [w444 w455]
            tunnel: [w444 w455] -> w405
            tunnel: w400 -> [w441 w452]
            tunnel: [_ FALSE ("Abort Parallel Computation")] -> w399
            tunnel: w398 -> [w440 w450]
            frame "Item 0", Default {
              # "Original fixed bin integration"
              n154 = Build Array(w447) -> (w439:T7[])
              n155 = call "Phasor Compute Gated Decay (Fixed Integration Steps).vi"("Non Dirac IRF or non-0 lifetime"=w441, "# Steps"=w442, "Error In"=w440, "IRF Period"=w445, "Gate & Decay Parameters Array"=w439, "Time Points {t_i}"=w446) -> ("Error Out"=w443:errorcluster, "{F(t_i)}"=w448:dbl[])  [unwired: 4 in]
            }
            frame "Item 1" {
              # "Modified VI-based numeric integration"
              n156 = Build Array(w458) -> (w449:T7[])
              n157 = call "Phasor Compute Gated Decay (Tolerance).vi"("Non Dirac IRF or non-0 lifetime"=w452, "tolerance"=w453, "Error In"=w450, "IRF Period"=w456, "Gate & Decay Parameters Array"=w449, "Time Points {t_i}"=w459) -> ("Error Out"=w451:errorcluster, "{F(t_i)}"=w457:dbl[])  [unwired: 4 in]
            }
          }
          n158 = global write "Phasor Abort Parallel Computation.vi" "Abort Parallel Computation"(w399) -> ()
          n159 = call "High Resolution Timing.vi"("relative seconds (NaN)"=w405) -> ("elapsed (relative) seconds"=w406:dbl)  [unwired: 16 in, 2 out]
        }
      }
    }
    frame True {
      # "Infinite number of gates"
      n160 = One Button Dialog(message="Can't compute an infinite number of gates, unless the gate is square, in which case an analytical approach is used...\nIn all other cases, use a finite number of gates (Settings>>Gates>># Gates).") -> ()  [unwired: 1 in, 1 out]
    }
  }
  "CPU (s)" <- w7
  n161 = expression code="W/2"(w28) -> (w51:ext)
  n162 = Compound Arithmetic op=MULTIPLY(w25, w46) -> (w3:ext[])
  n163 = case shown="False" w1 {
    tunnel: w3 -> [w468 w470]
    tunnel: [w468 w469] -> w2
    frame False {
    }
    frame True {
      n164 = call "Poisson Randomize Array.vi"("Array"=w470) -> ("Poisson Randomized Array"=w469:dbl[])  [unwired: 10 in]
    }
  }
  n165 = Array Max & Min(array=w25) -> (max value=w29:ext)  [unwired: 3 out]
  n166 = Select(t=w51, s=w48, f=ext 0.0 ("t")) -> (s? t:f=w53:ext)
  n167 = call "Phasor Compute Saturated Gate Image Array.vi"("error in (no error)"=w14, "Saturation Parameters"=w40, "Gate Count Rate Array in"=w2) -> ("error out"=→"Error Out":errorcluster, "Saturated Gate Image Count Array out"=w37:ext[])  [unwired: 7 in]
  n168 = Less Or Equal?(x=w29, y=ext 1.0842021724855044e-19) -> (x <= y?=→"Small Gate Values?":bool)
  n169 = Compound Arithmetic op=ADD(w53, w24) -> (w19:ext[])
  "t Array" <- w19
  n170 = Array Max & Min(array=w37) -> (max value=w18:ext)  [unwired: 3 out]
  n171 = Select(t=w18, s=w36, f=ext 1.0) -> (s? t:f=w35:ext)
  n172 = Compound Arithmetic op=MULTIPLY(invert w35, w37) -> (w17:ext[])
  "Gate Image Array" <- w17
  n173 = disable-structure shown="Enabled" {
    disable-tunnel: w19 -> [w474 _]
    disable-tunnel: w17 -> [w471 _]
    frame Disabled {
      n174 = Bundle(w474, w471) -> (w472:cluster{ext[], ext[]})  [unwired: 1 in]
      n175 = Build Array(w472) -> (→"XY Graph":cluster{ext[], ext[]}[])
    }
    frame Enabled {
    }
  }
